vi "Pre Launch Init.vi"(11 "Gui in":refnum<class "Gui.lvclass">) -> (0 "error out":errorcluster, 3 "Gui out":refnum<class "Gui.lvclass">)   [LabVIEW 2022 SP3, in "Gui.lvlib" / "Gui.lvclass"]
doc: "(<B>Filename</B>: Actor Framework.lvlib:Actor.lvclass:Pre Launch Init.vi)\n\nDefines behavior that occurs after the Launch Actor method is invoked but before the actor's Actor Core method begins running.\n\nThe Pre Launch Init method is guaranteed to finish before the Launch Actor method returns to its caller and before the actor itself receives any messages. Any references that the Pre Launch Init method obtains are guaranteed to have the same lifetime as the actor itself. Any errors that the Pre Launch Init method returns will abort the launch.\n\nBy default, this method does nothing. A descendant class may override it to define behavior."
uses:
  Gui.lvclass
  Gui.lvclass/Gui.ctl
  <vilib>/ActorFramework/Actor/Actor.lvclass
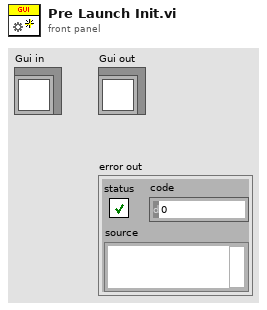
[diagram p1: front panel]
types:
  T1 = typedef "Gui.lvlib/Gui.lvclass/_Events.ctl" = cluster{"StopGuiLoop":refnum<user-event>}
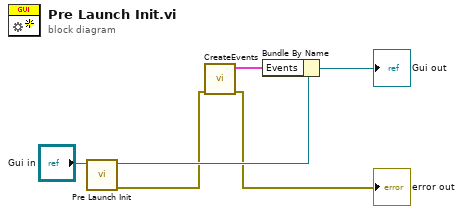
[diagram p0: block diagram]
diagram:
  n1 = call-parent "Pre Launch Init.vi"("Actor in"="Gui in") -> ("error out"=w1:errorcluster, "Actor out"=w5:refnum<class "Gui.lvclass">)  [unwired: 9 in]
  n2 = call "CreateEvents.vi"("error in (no error)"=w1) -> ("error out"=→"error out":errorcluster, "Events"=w2:T1)  [unwired: 9 in]
  n3 = Bundle By Name(cluster=w5, "Events"=w2) -> (→"Gui out":refnum<class "Gui.lvclass">)
